vi "Winch_MRay.vi"(8 "Setpoints":dbl[](array[numeric]), 9 "Buttons":T1, 10 "Current POT":dbl format="%#_13g", 11 "Winch State":i32) -> (1 "Winch Out":dbl, 3 "Winch State":i32)   [LabVIEW 2013]
uses:
  <vilib>/Rock Robotics/WPI/Joystick/WPI_JoystickButtonState.ctl
panel:
  in  "BallTrigger":bool
  out "Shoot Ready":bool
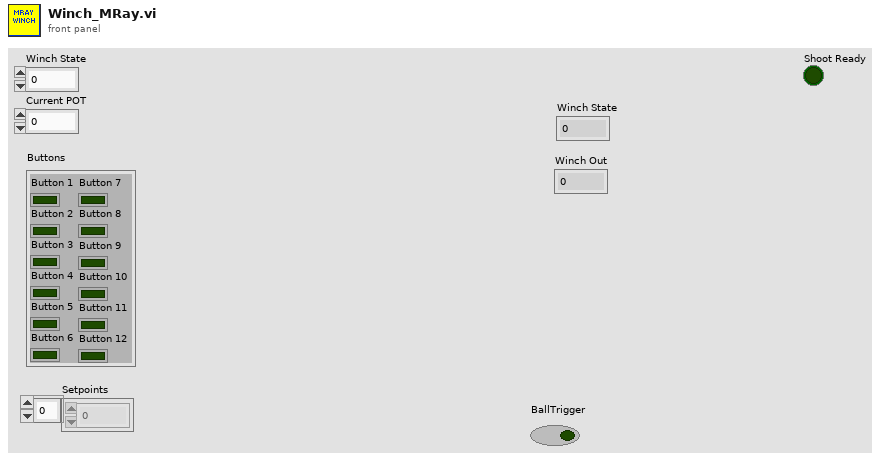
[diagram p1: front panel]
types:
  T1 = typedef "WPI_JoystickButtonState.ctl" = cluster{"Button 1":bool, "Button 2":bool, "Button 3":bool, "Button 4":bool, "Button 5":bool, "Button 6":bool, "Button 7":bool, "Button 8":bool, "Button 9":bool, "Button 10":bool, "Button 11":bool, "Button 12":bool}
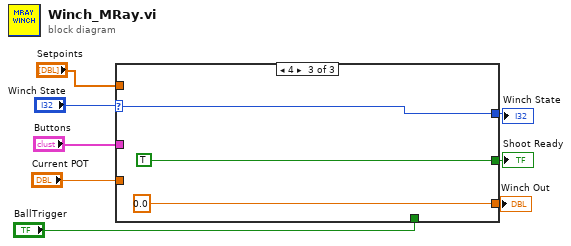
[diagram p0: block diagram]
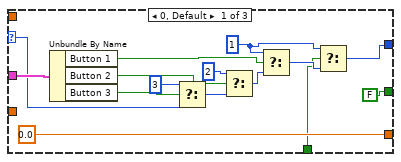
[diagram p2: hidden frame]
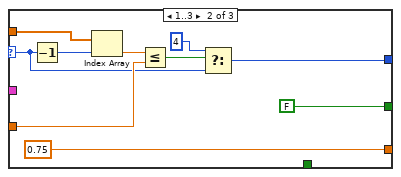
[diagram p3: hidden frame]
diagram:
  n1 = case shown="4" "Winch State" {
    selector: "Winch State" -> [w22 w27 w34]
    tunnel: "Setpoints" -> [_ w32 _]
    tunnel: "Buttons" -> [w23 _ _]
    tunnel: [w10 w26 w34] -> w5
    tunnel: [0.0 ("t") 0.75 ("t") 0.0 ("t")] -> w4
    tunnel: "Current POT" -> [_ w31 _]
    tunnel: [FALSE FALSE TRUE] -> w2
    tunnel: "BallTrigger" -> [w11 _ _]
    frame 0, Default {
      w9 = 1 ("t")
      n2 = Unbundle By Name(w23) -> ("Button 1"=w17:bool, "Button 2"=w16:bool, "Button 3"=w15:bool)
      n3 = Select(t=3, s=w15, f=w22) -> (s? t:f=w20:i32)
      n4 = Select(t=2, s=w16, f=w20) -> (s? t:f=w18:i32)
      n5 = Select(t=w9, s=w17, f=w18) -> (s? t:f=w12:i32)
      n6 = Select(t=w9, s=w11, f=w12) -> (s? t:f=w10:i32)
    }
    frame 1..3 {
      n7 = Decrement(x=w27) -> (x-1=w33:i32)
      n8 = Index Array(array=w32, index=w33) -> (element=w30:dbl)
      n9 = Less Or Equal?(x=w30, y=w31) -> (x <= y?=w29:bool)
      n10 = Select(t=4, s=w29, f=w27) -> (s? t:f=w26:i32)
    }
    frame 4 {
    }
  }
  "Winch State" <- w5
  "Winch Out" <- w4
  "Shoot Ready" <- w2
